vi "GetHelp.vi"(11 "DiscoverTestCases in":refnum<class "DiscoverTestCases.lvclass">) -> (2 "Help out":string, 3 "DiscoverTestCases out":refnum<class "DiscoverTestCases.lvclass">)   [LabVIEW 2027, in "DiscoverTestCases.lvclass"]
uses:
  DiscoverTestCases.lvclass
panel:
  in  "Help in":string="LabVIEWCLI -OperationName DiscoverTestCases  -RepositoryPath <path to repository>\n\n -RepositoryPath  The path to the repository on disk to scan for test cases."
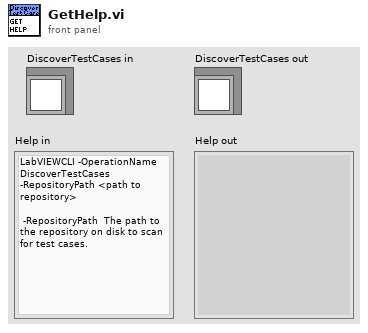
[diagram p1: front panel]
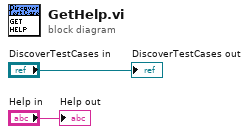
[diagram p0: block diagram]
diagram:
  "Help out" <- "Help in"
  "DiscoverTestCases out" <- "DiscoverTestCases in"
